vi "No_Change.vi"(9 "Field and Tep  Range":T1, 10 "ScanQ in":refnum<queue>, 11 "Queue in":refnum<queue>) -> (2 "ScanQ out":refnum<queue>, 3 "Queue out":refnum<queue>)   [LabVIEW 2025]
uses:
  STM-Auto-Project/QMH CTLS/Sweeper.ctl
  STM-Auto-Project/QMH CTLS/Scan_Params (QMH).ctl
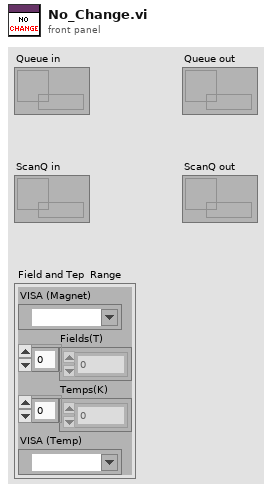
[diagram p1: front panel]
types:
  T1 = cluster{"VISA (Magnet)":refnum<visa-resource-name>, "Fields(T)":dbl[], "Temps(K)":dbl[], "VISA (Temp) ":refnum<visa-resource-name>}
  T2 = enum16{"1. BIAS", "2. INIT_SCAN", "3. SCAN_IDLE", "4. INTER_SCAN", "5. NEW_COORDS_&_FRAME", "6. FINAL_SCAN", "7. POLL BIAS ", "8. STOP"}
  T3 = typedef "Scan_Params (QMH).ctl" = cluster{"Setpoint (I)":dbl[], "Bias (V)":dbl[], "Number of scans":u8, "Port number (3364)":u32, "Avoid zero threshold (V)":dbl, "Current State":enum16{"1. BIAS", "2. INIT_SCAN", "3. SCAN_IDLE", "4. INTER_SCAN", "5. NEW_COORDS_&_FRAME", "6. FINAL_SCAN", "7. POLL BIAS ", "8. STOP"}}
  T4 = enum16{"NO CHANGE", "SET TEMP & FIELD", "SWEEP IDLE", "NEXT TEMP & FIELD", "SWEEP DONE"}
  T5 = typedef "Sweeper.ctl" = cluster{"Temps(K)":dbl[], "Fields(T)":dbl[], "Sweep States":enum16{"NO CHANGE", "SET TEMP & FIELD", "SWEEP IDLE", "NEXT TEMP & FIELD", "SWEEP DONE"}}
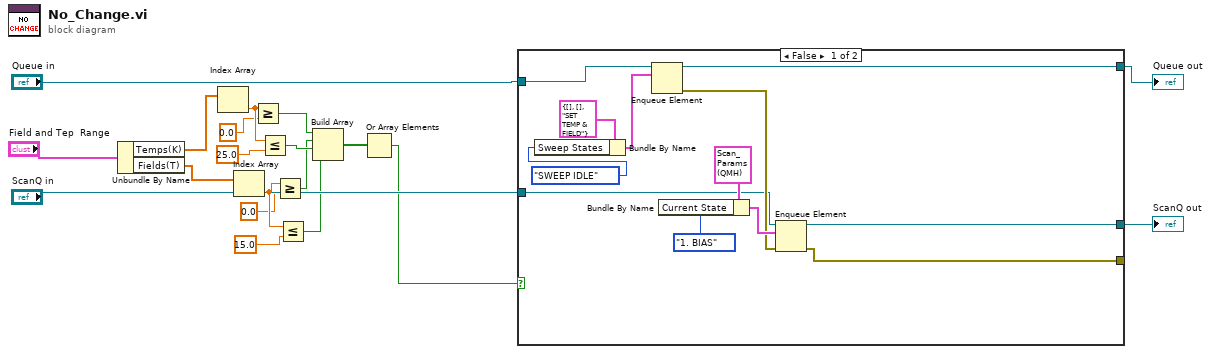
[diagram p0: block diagram]
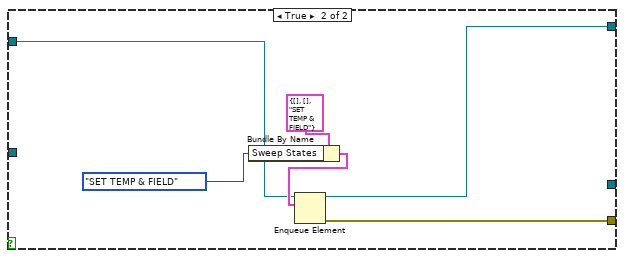
[diagram p2: hidden frame]
diagram:
  n1 = Unbundle By Name("Field and Tep  Range") -> ("Temps(K)"=w2:dbl[], "Fields(T)"=w1:dbl[])
  n2 = Index Array(array=w2) -> (element=w13:dbl)  [unwired: 1 in]
  n3 = Index Array(array=w1) -> (element=w9:dbl)  [unwired: 1 in]
  n4 = Greater Or Equal?(x=w13, y=0.0) -> (x >= y?=w5:bool)
  n5 = Less Or Equal?(x=w13, y=25.0) -> (x <= y?=w12:bool)
  n6 = Greater Or Equal?(x=w9, y=0.0) -> (x >= y?=w6:bool)
  n7 = Less Or Equal?(x=w9, y=15.0) -> (x <= y?=w11:bool)
  n8 = Build Array(w5, w6, w12, w11) -> (w8:bool[])
  n9 = Or Array Elements(Boolean array=w8) -> (logical OR=w7:bool)
  n10 = case shown="False" w7 {
    tunnel: [w25 w35] -> w18
    tunnel: [w23 w34] -> _
    tunnel: [w26 _] -> w19
    tunnel: "Queue in" -> [w22 w32]
    tunnel: "ScanQ in" -> [w20 _]
    frame False {
      n11 = Bundle By Name(cluster=T5 {"Temps(K)"=[], "Fields(T)"=[], "Sweep States"=enum."SET TEMP & FIELD"} ("element"), "Sweep States"=T4."SWEEP IDLE") -> (w29:T5)
      n12 = Enqueue Element(queue=w22, element=w29) -> (queue out=w25:refnum<queue>, error out=w24:errorcluster)  [unwired: 2 in, 1 out]
      n13 = Bundle By Name(cluster=T3 {"Setpoint (I)"=[], "Bias (V)"=[], "Number of scans"=1, "Port number (3364)"=3364, "Avoid zero threshold (V)"=0.004999999888241291, "Current State"=enum."1. BIAS"} ("element"), "Current State"=T2."1. BIAS") -> (w27:T3)
      n14 = Enqueue Element(queue=w20, element=w27, error in (no error)=w24) -> (queue out=w26:refnum<queue>, error out=w23:errorcluster)  [unwired: 1 in, 1 out]
    }
    frame True {
      n15 = Bundle By Name(cluster=T5 {"Temps(K)"=[], "Fields(T)"=[], "Sweep States"=enum."SET TEMP & FIELD"} ("element"), "Sweep States"=T4."SET TEMP & FIELD") -> (w36:T5)
      n16 = Enqueue Element(queue=w32, element=w36) -> (queue out=w35:refnum<queue>, error out=w34:errorcluster)  [unwired: 2 in, 1 out]
    }
  }
  "ScanQ out" <- w19
  "Queue out" <- w18
